vi "SetSettings.vi"(8 "error in (no error)":errorcluster, 10 "Variant":variant, 11 "ChromaAcLoad in":refnum<class "ChromaAcLoad.lvclass">) -> (0 "error out":errorcluster, 3 "ChromaAcLoad Out":refnum<class "ChromaAcLoad.lvclass">)   [LabVIEW 2018, in "AcPwrPlugins.lvlib" / "ChromaAcLoad.lvclass"]
doc: "This VI retrieves a boolean status to see if the instrument can conduct measurements while the device is changing modes or turning off and on."
uses:
  ChromaAcLoad.lvclass
  C:/Users/ico/Documents/Projects/NistPluggableModules/AcPwr/AcPwrPlugins/AcPwrBaseClass/AcPwrBase.lvclass
  AcPwrBaseClass/AcPwrBase.lvclass/AcPwrBase.ctl
  AcPwrBaseClass/Accessors/Read BaseMeasurements.vi
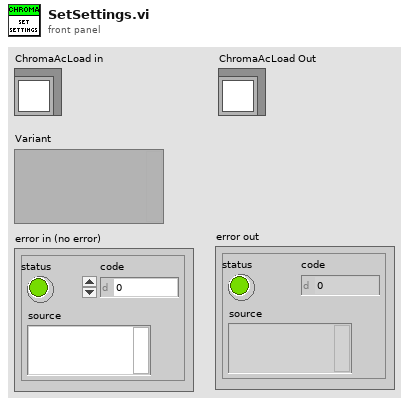
[diagram p1: front panel]
types:
  T1 = typedef "AcPwrPlugins.lvlib/ChromaAcLoad.lvclass/DeviceProperties.ctl" = cluster{"Configuration Mode":enum16{"Constant Voltage (DC)", "Constant Power (DC)", "Constant Power (AC)", "Constant Current (DC)", "Constant Current (AC)", "Constant Resistance (DC)", "Constant Resistance (AC)", "Rectified Mode (DC)", "Inrush (AC)", "RLC CP (AC)", "RLC (AC)"}, "Phases":cluster{"Handle":string, "Name":string, "Phase Select":i32, "Instrument Options":string, "id query (T)":bool, "reset device (T)":bool, "Load Short Circuited":bool, "Line Synchronization":bool, "Load Current (A/Arms)":dbl, "Load Voltage (V/Vrms)":dbl, "Load Power (W)":dbl, "Load Resistance (Ohms)":dbl, "Load Current Peak Limit (A)":dbl, "Load Current Limit (A/Arms)":dbl, "Load Power Limit (W)":dbl, "Synch Frequency (Hz)":dbl, "Priority":enum16{"CF Only", "PF Only", "Both (CF)", "Both (PF)"}, "Crest Factor":dbl, "Power Factor":dbl, "Slew Rate":cluster{"Rise Slew Rate (A/ms)":i32, "Fall Slew Rate (A/ms)":i32}, "LC/RLC Mode":cluster{"Capacitance (uF)":i32, "Inductance (uH)":i32, "Series Resistance (Ohm)":dbl, "Parallel Resistance (Ohm)":dbl}, "Timing":cluster{"TimingOn":enum16{""}, "Hours":u32, "Minutes":u32, "Seconds":dbl, "CutoffVoltage":dbl}, "Connected":bool}[]}
  T2 = typedef "AcPwrPlugins.lvlib/AcPwrBase.lvclass/BaseMeasurements.ctl" = cluster{"Handle":string, "Name":string, "Enabled":bool, "Measurement Value":dbl, "btnMeasFetch":bool, "Chroma Hold Peak Current Measurement":bool, "Chroma Measurement Type":T3, "Chroma Protection Status String":string, "NHRDC Fetch Method":i32, "NHRDC Fetch Time (s)":sgl, "NHRDC Measurement Type":i32, "NHRGridSim Measurement Type ":enum16{"Average Current", "Max Current", "Min Current", "Average Voltage", "Max Voltage", "Min Voltage", "Average True Power", "Max True Power", "Min True Power", "Average Apparent Power", "Max Apparent Power", "Min Apparent Power", "Power Factor", "Crest Factor"}, "NHRGridSim Phase ":i32, "PPS Measurement Type ":enum16{"Voltage RMS L-N", "Voltage RMS L-L", "Frequency", "Current RMS", "Current Peak", "Crest Factor", "Power Factor", "Power VA", "Real Power"}, "PPS Channel Name":enum16{"A", "B", "C"}}[]
  T3 = typedef "AcPwrPlugins.lvlib/ChromaAcLoad.lvclass/MeasurementType.ctl" = enum16{"Voltage (Vrms or V)", "Current (Arms or A)", "Power (W)", "Peak Voltage (V)", "Peak Current (A)", "Peak Power (W)", "Frequency (Hz)", "Resistance (Ohms)", "Voltage Overshoot (V)", "Positive Peak Current (A)", "Voltage Undershoot (V)", "Negative Peak Current (A)", "Apparent Power (VA)", "Reacitive Power (VAR)", "Voltage THD", "Power Factor", "Current's Crest Factor"}
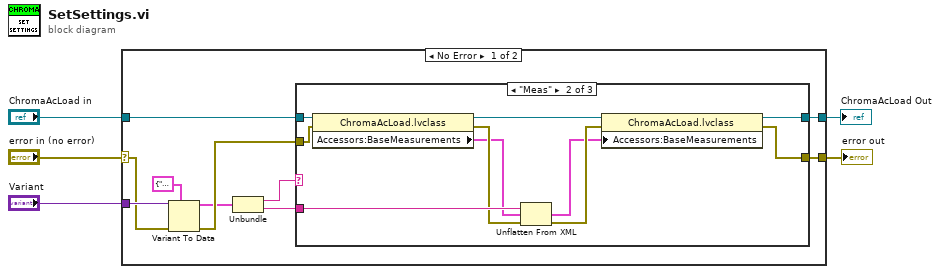
[diagram p0: block diagram]
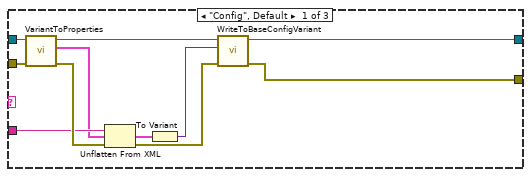
[diagram p2: hidden frame]
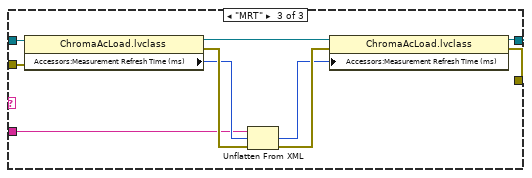
[diagram p3: hidden frame]
diagram:
  n1 = case shown="No Error" "error in (no error)" {
    selector: "error in (no error)" -> [w11 w48]
    tunnel: [w14 w48] -> w4
    tunnel: "ChromaAcLoad in" -> [w15 w47]
    tunnel: "Variant" -> [w12 _]
    tunnel: [w13 w47] -> w1
    frame No Error {
      n2 = Variant To Data(error in=w11, type=cluster{string, string} {"", ""}, Variant=w12) -> (data=w8:cluster{string, string}, error out=w9:errorcluster)
      n3 = Unbundle(w8) -> (w6:string, w7:string)
      n4 = case shown="\"Meas\"" w6 {
        tunnel: [w19 w36 w37] -> w14
        tunnel: w15 -> [w21 w32 w41]
        tunnel: [w16 w35 w38] -> w13
        tunnel: w9 -> [w26 w31 w40]
        tunnel: w7 -> [w24 w33 w39]
        frame "Config", Default {
          n5 = call "VariantToProperties.vi"("error in (no error)"=w26, "ChromaAcLoad"=w21) -> ("error out"=w25:errorcluster, "Device Properties"=w22:T1, "ChromaAcLoad"=w17:refnum<class "ChromaAcLoad.lvclass">)  [unwired: 7 in]
          n6 = Unflatten From XML(xml string=w24, type=w22, error in (no error)=w25) -> (value=w23:T1, error out=w20:errorcluster)
          n7 = To Variant(anything=w23) -> (Variant=w18:variant)
          n8 = call "WriteToBaseConfigVariant.vi"("error in (no error)"=w20, "Variant"=w18, "ChromaAcLoad in"=w17) -> ("error out"=w19:errorcluster, "ChromaAcLoad out"=w16:refnum<class "ChromaAcLoad.lvclass">)  [unwired: 7 in]
        }
        frame "Meas" {
          n9 = property class="ChromaAcLoad.lvclass"(reference=w32, error in=w31) -> (reference out=w29:refnum<class "ChromaAcLoad.lvclass">, error out=w30:errorcluster, "Accessors:BaseMeasurements"=w28:T2)
          n10 = Unflatten From XML(xml string=w33, type=w28, error in (no error)=w30) -> (value=w27:T2, error out=w34:errorcluster)
          n11 = property class="ChromaAcLoad.lvclass"(reference=w29, error in=w34, "Accessors:BaseMeasurements"=w27) -> (reference out=w35:refnum<class "ChromaAcLoad.lvclass">, error out=w36:errorcluster)
        }
        frame "MRT" {
          n12 = property class="ChromaAcLoad.lvclass"(reference=w41, error in=w40) -> (reference out=w44:refnum<class "ChromaAcLoad.lvclass">, error out=w45:errorcluster, "Accessors:Measurement Refresh Time (ms)"=w43:u32)
          n13 = Unflatten From XML(xml string=w39, type=w43, error in (no error)=w45) -> (value=w42:u32, error out=w46:errorcluster)
          n14 = property class="ChromaAcLoad.lvclass"(reference=w44, error in=w46, "Accessors:Measurement Refresh Time (ms)"=w42) -> (reference out=w38:refnum<class "ChromaAcLoad.lvclass">, error out=w37:errorcluster)
        }
      }
    }
    frame Error {
    }
  }
  "error out" <- w4
  "ChromaAcLoad Out" <- w1
